vi "BRig_Host_dataRunState_typeStart.vi"(5 "input_nTrial":u16, 7 "input_LorR":u16, 9 "input_idx":i32[](array[numeric]), 10 "input_dataTS":u16[][](array[numeric]), 11 "input_dataPlot":u16[][](array[numeric])) -> (1 "output_idx":i32[](array[numeric]), 2 "output_dataTS":u16[][](array[numeric]), 3 "output_dataPlot":u16[][](array[numeric]), 4 "output_updatePlot":bool)   [LabVIEW 2014]
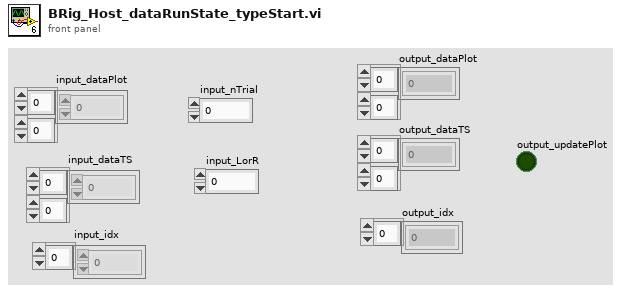
[diagram p1: front panel]
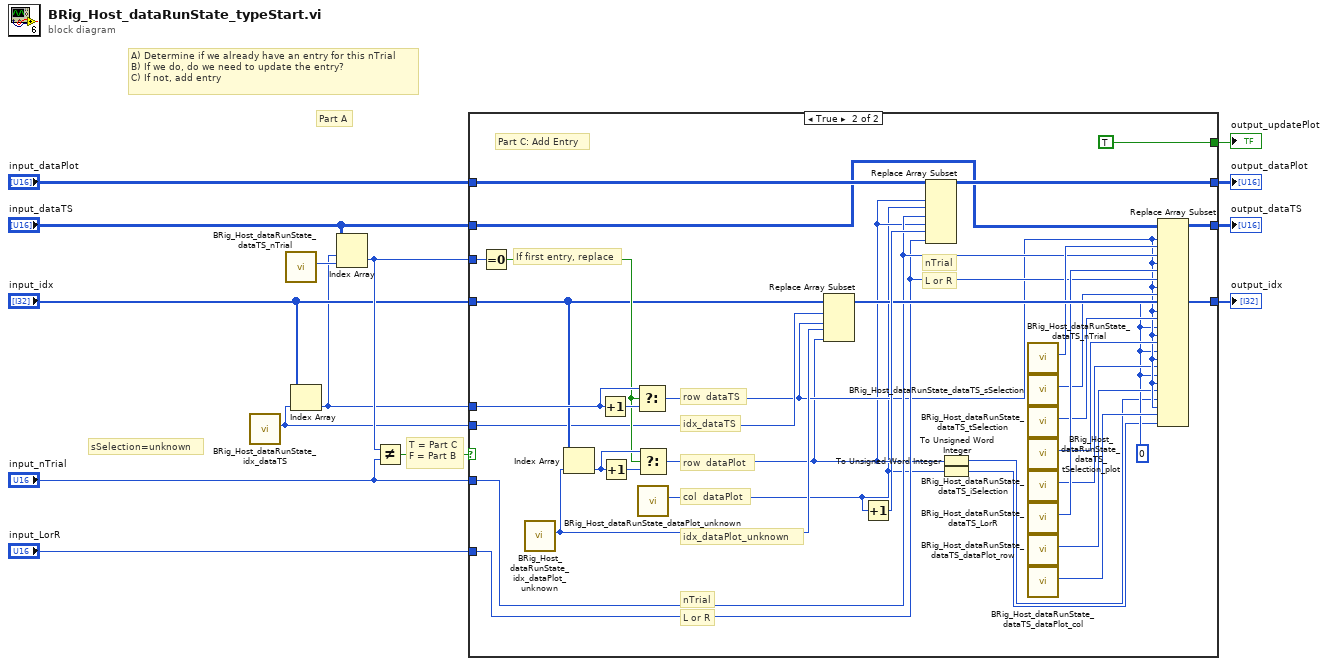
[diagram p0: block diagram]
diagram:
  # "T = Part C\nF = Part B"
  # "Part A"
  # "A) Determine if we already have an entry for this nTrial\nB) If we do, do we need to update the entry?\nC) If not, add entry"
  # "sSelection=unknown"
  n1 = call "BRig_Host_dataRunState_idx_dataTS.vi"() -> ("output_idx_dataTS"=w6:i32)  [unwired: 11 in]
  n2 = call "BRig_Host_dataRunState_dataTS_nTrial.vi"() -> ("output_idx_dataTS_nTrial"=w14:i32)  [unwired: 11 in]
  n3 = Index Array(array="input_idx", index=w6) -> (element=w7:i32)
  n4 = Index Array(array="input_dataTS", index (row)=w7, index (col)=w14) -> (element=w12:u16)
  n5 = Not Equal?(x=w12, y="input_nTrial") -> (x != y?=w13:bool)
  n6 = case shown="True" w13 {
    tunnel: w12 -> [_ w49]
    tunnel: "input_dataTS" -> [w16 w39]
    tunnel: "input_LorR" -> [_ w31]
    tunnel: "input_nTrial" -> [_ w33]
    tunnel: "input_idx" -> [w15 w38]
    tunnel: w7 -> [_ w47]
    tunnel: w6 -> [_ w37]
    tunnel: "input_dataPlot" -> [w17 w43]
    tunnel: [w17 w41] -> w4
    tunnel: [w16 w40] -> w3
    tunnel: [w15 w35] -> w2
    tunnel: [_ TRUE] -> w1
    frame False {
      # "Ignore for now"
      # "Part B: Do we need to update the entry?"
    }
    frame True {
      w23 = u16 0 ("new element/subarray")
      # "L or R"
      # "nTrial"
      # "L or R"
      # "nTrial"
      # "col  dataPlot"
      # "idx_dataPlot_unknown"
      # "row  dataPlot"
      # "row  dataTS"
      # "idx_dataTS"
      # "If first entry, replace"
      # "Part C: Add Entry"
      n7 = Equal To 0?(x=w49) -> (x = 0?=w44:bool)
      n8 = call "BRig_Host_dataRunState_idx_dataPlot_unknown.vi"() -> ("output_idx_dataPlot_unknown"=w36:i32)  [unwired: 11 in]
      n9 = Index Array(array=w38, index=w36) -> (element=w45:i32)
      n10 = Increment(x=w47) -> (x+1=w48:i32)
      n11 = Increment(x=w45) -> (x+1=w46:i32)
      n12 = Select(t=w47, s=w44, f=w48) -> (s? t:f=w27:i32)
      n13 = Select(t=w45, s=w44, f=w46) -> (s? t:f=w21:i32)
      n14 = call "BRig_Host_dataRunState_dataPlot_unknown.vi"() -> ("output_idx_dataPlot_unknown"=w19:i32)  [unwired: 11 in]
      n15 = Replace Array Subset(array=w38, new element #1=w27, index #1=w37, new element #2=w21, index #2=w36) -> (w35:i32[])
      n16 = Increment(x=w19) -> (x+1=w42:i32)
      n17 = Replace Array Subset(array=w43, new element #1=w33, index (row) #1=w21, index (col) #1=w19, new element #2=w31, index (row) #2=w21, index (col) #2=w42) -> (w41:u16[][])
      n18 = To Unsigned Word Integer(number=w21) -> (unsigned 16bit integer=w20:u16)
      n19 = To Unsigned Word Integer(number=w19) -> (unsigned 16bit integer=w18:u16)
      n20 = call "BRig_Host_dataRunState_dataTS_nTrial.vi"() -> ("output_idx_dataTS_nTrial"=w34:i32)  [unwired: 11 in]
      n21 = call "BRig_Host_dataRunState_dataTS_sSelection.vi"() -> ("output_idx_dataTS_sSelection"=w30:i32)  [unwired: 11 in]
      n22 = call "BRig_Host_dataRunState_dataTS_tSelection.vi"() -> ("output_idx_dataTS_tSelection"=w29:i32)  [unwired: 11 in]
      n23 = call "BRig_Host_dataRunState_dataTS_tSelection_plot.vi"() -> ("output_idx_dataTS_tSelection_plot"=w28:i32)  [unwired: 11 in]
      n24 = call "BRig_Host_dataRunState_dataTS_iSelection.vi"() -> ("output_idx_dataTS_iSelection"=w26:i32)  [unwired: 11 in]
      n25 = call "BRig_Host_dataRunState_dataTS_LorR.vi"() -> ("output_idx_dataTS_LorR"=w32:i32)  [unwired: 11 in]
      n26 = call "BRig_Host_dataRunState_dataTS_dataPlot_row.vi"() -> ("output_idx_dataTS_dataPlot_row"=w25:i32)  [unwired: 11 in]
      n27 = call "BRig_Host_dataRunState_dataTS_dataPlot_col.vi"() -> ("output_idx_dataTS_dataPlot_col"=w24:i32)  [unwired: 11 in]
      n28 = Replace Array Subset(array=w39, new element #1=w33, index (row) #1=w27, index (col) #1=w34, new element #2=w31, index (row) #2=w27, index (col) #2=w32, new element #3=w23, index (row) #3=w27, index (col) #3=w30, new element #4=w23, index (row) #4=w27, index (col) #4=w29, new element #5=w23, index (row) #5=w27, index (col) #5=w28, new element #6=w23, index (row) #6=w27, index (col) #6=w26, new element #7=w20, index (row) #7=w27, index (col) #7=w25, new element #8=w18, index (row) #8=w27, index (col) #8=w24) -> (w40:u16[][])
    }
  }
  "output_dataPlot" <- w4
  "output_dataTS" <- w3
  "output_idx" <- w2
  "output_updatePlot" <- w1
